vi "LINX - Live reset.vi"() -> ()   [LabVIEW 2019]
uses:
  vi.lib/LINXx/Public/Reset Target.ctl
  <vilib>/MakerHub/LINX/Public/Utilities/Open Serial.vi
  <vilib>/MakerHub/LINX/LMH-LINX.lvlib
  vi.lib/LINXx/LINXx.lvlib
panel:
  out "Loop Rate (Hz)":u32
  in  "stop":bool
  in  "Serial Port":refnum<visa-resource-name>="N/A"
  in  "Reset":bool
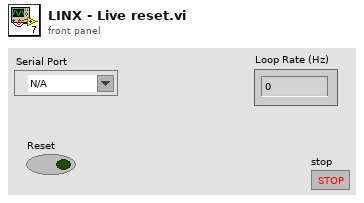
[diagram p1: front panel]
types:
  T1 = typedef "LMH-LINX.lvlib/LINX Ref.ctl" = cluster{"IO":T2, "Interface":T3, "LINX Device Config":T4}
  T2 = typedef "LMH-LINX.lvlib/Platform.ctl" = enum16{"Remote", "Local"}
  T3 = typedef "LMH-LINX.lvlib/Interface.ctl" = enum16{"Serial", "TCP"}
  T4 = typedef "LMH-LINX.lvlib/Device.lvlib/LINX Device Config.ctl" = cluster{"Interface":T3, "COM Port":refnum<visa-resource-name>, "TCP Configuration":T5, "Device Family":u8, "Device ID":u8, "Device Name":string, "TCP Ref":refnum<k5>, "Channels":T6}
  T5 = typedef "LMH-LINX.lvlib/Device.lvlib/TCP Config.ctl" = cluster{"IP Address":string, "Port":u16}
  T6 = typedef "LMH-LINX.lvlib/Channels.ctl" = cluster{"DI":u8[], "DO":u8[], "AI":u8[], "AO":u8[], "PWM":u8[], "QE":u8[], "UART":u8[], "I2C 2":u8[], "SPI":u8[], "CAN":u8[], "Servo":u8[], "AI Ref (V)":dbl, "AI Resolution (Bits)":u8, "AO Ref (V)":dbl, "AO Resolution (Bits)":u8}
  T7 = typedef "LINXx.lvlib/Reset Target.ctl" = enum16{"None", "Serial", "TCP", "Board"}
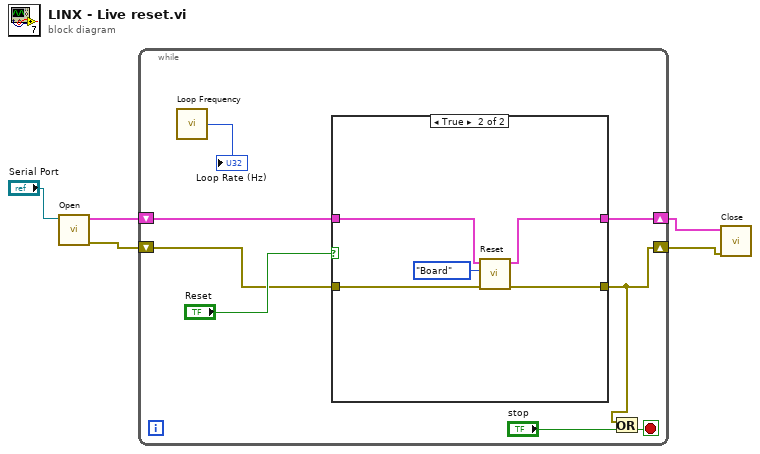
[diagram p0: block diagram]
diagram:
  n1 = call-poly <vilib>:"Open.vi"("Serial Port"="Serial Port") -> ("Error Out"=w4:errorcluster, "LINX Resource"=w5:T1)  [unwired: 8 in, 1 out]
  n2 = while {
    shift-right: [w11] -> w3
    shift-left: w5 -> [w12]
    shift-right: [w7] -> w2
    shift-left: w4 -> [w10]
    stop <- w8 stop-if-true
    n3 = call <vilib>:"Loop Frequency.vi"() -> ("Loop Rate (Hz)"=→"Loop Rate (Hz)":u32)
    n4 = case shown="True" "Reset" {
      tunnel: w12 -> [w15 w20]
      tunnel: [w15 w19] -> w11
      tunnel: [w14 w18] -> w7
      tunnel: w10 -> [w14 w17]
      frame False {
      }
      frame True {
        n5 = call "Reset.vi"("Error In"=w17, "Reset Target"=Reset_Target."Board", "LINX Resource"=w20) -> ("Error Out"=w18:errorcluster, "LINX Resource out"=w19:T1)  [unwired: 7 in]
      }
    }
    n6 = Or(x=w7, y="stop") -> (x .or. y?=w8:bool)
  }
  n7 = call <vilib>:"Close.vi"("Error In"=w2, "LINX Resource"=w3) -> ()  [unwired: 9 in, 1 out]
